vi "Core Actor - Init User Events.vi"(8 "error in (no error)":errorcluster, 11 "Child_2_Class in":refnum<class "Child_2_Class.lvclass">=refnum) -> (0 "error out":errorcluster, 3 "Child_2_Class out":refnum<class "Child_2_Class.lvclass">)   [LabVIEW 2023, in "Actor_Child_2.lvlib" / "Child_2_Class.lvclass"]
uses:
  Child_2_Class.lvclass
  Usr Ev/Child_2 - Ctrl - Action.ctl
  <vilib>/ActorFramework/Actor/Actor.lvclass
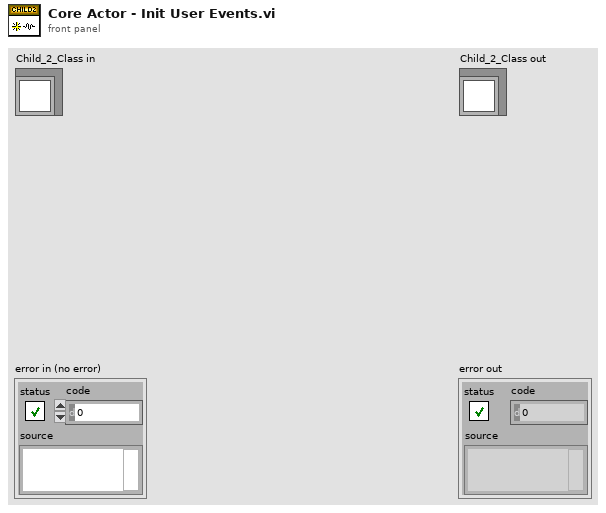
[diagram p1: front panel]
types:
  T1 = typedef "Actor_Child_2.lvlib/Child_2_Class.lvclass/Child_2 - Ctrl - Action.ctl" = enum16{"Reg Ev", "Get Refs", "Close Ev", "Populate Enum with Events"}
  T2 = typedef "Actor_Child_2.lvlib/Child_2_Class.lvclass/Child_2 - Ctrl - Usr Ev Ref.ctl" = cluster{"SEND MESSAGE Ev":cluster{"Data":refnum<user-event>}, "STOP_ACTOR Ev":cluster{"Data":refnum<user-event>}, "INIT_ACTOR Ev":cluster{"Data":refnum<user-event>}, "START Ev":cluster{"Data":refnum<user-event>}, "STOP Ev":cluster{"Data":refnum<user-event>}, "GET Ev":cluster{"Data":refnum<user-event>}, "SET Ev":cluster{"Data":refnum<user-event>}, "ERROR_HANDLER Ev":cluster{"Data":refnum<user-event>}, "RESET Ev":cluster{"Data":refnum<user-event>}, "T2 Ev":cluster{"Data":refnum<user-event>}, "T3 Ev":cluster{"Data":refnum<user-event>}, "T4 Ev":cluster{"Data":refnum<user-event>}}
  T3 = typedef "Actor_Child_2.lvlib/Child_2_Class.lvclass/Child_2 - Ctrl - Usr Ev Reg - Refs.ctl" = cluster{"ERR1":refnum<event-registration>, "ERR2":refnum<event-registration>, "ERR3":refnum<event-registration>, "ERR4":refnum<event-registration>, "ERR5":refnum<event-registration>}
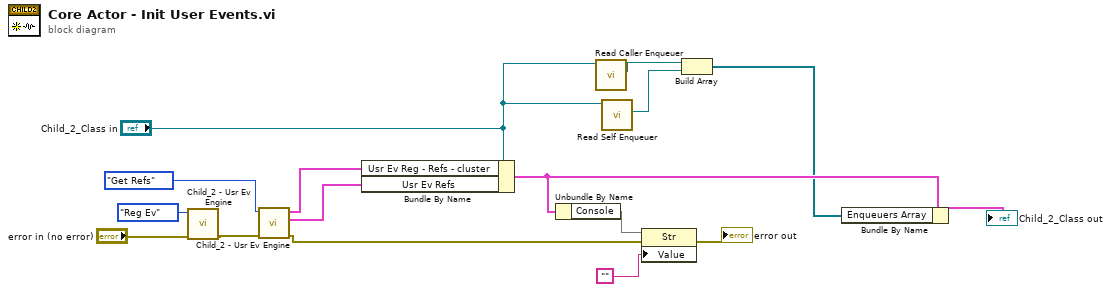
[diagram p0: block diagram]
diagram:
  n1 = call "Child_2 - Usr Ev Engine.vi"("error in (no error)"="error in (no error)", "Action"=Child_2_-_Ctrl_-_Action."Reg Ev") -> ("error out"=w15:errorcluster)  [unwired: 6 in, 3 out]
  n2 = call "Child_2 - Usr Ev Engine.vi"("error in (no error)"=w15, "Action"=Child_2_-_Ctrl_-_Action."Get Refs") -> ("error out"=w8:errorcluster, "Usr Ev Refs"=w11:T2, "Usr Ev Reg - Refs - cluster"=w12:T3)  [unwired: 6 in, 1 out]
  n3 = Bundle By Name(cluster="Child_2_Class in", "Usr Ev Reg - Refs - cluster"=w12, "Usr Ev Refs"=w11) -> (w6:cluster{})
  n4 = Unbundle By Name(w6) -> ("Console"=w10)
  n5 = call <vilib>:"Read Caller Enqueuer.vi"("Actor"="Child_2_Class in") -> ("Caller Enqueuer"=w5:refnum<class "Message Enqueuer.lvclass">)  [unwired: 10 in]
  n6 = call <vilib>:"Read Self Enqueuer.vi"("Actor"="Child_2_Class in") -> ("Self Enqueuer"=w4:refnum<class "Message Enqueuer.lvclass">)  [unwired: 10 in]
  n7 = property class="Str"(reference=w10, error in=w8, "Value"="") -> (error out=→"error out":errorcluster)  [unwired: 1 out]
  n8 = Build Array(w5, w4) -> (w2:refnum<class "Message Enqueuer.lvclass">[])
  n9 = Bundle By Name(cluster=w6, "Enqueuers Array"=w2) -> (→"Child_2_Class out":cluster{})
